vi "Autonomous Independent.vi"() -> ()   [LabVIEW 2014]
doc: "This VI is called when autonomous begins, and will automatically be terminated when autonomous ends. You can carry out timed or sensor driven robot movement independently without needing to return to the caller."
uses:
  <vilib>/Rock Robotics/WPI/Joystick/WPI_JoystickGetSetRefNum.vi
  <vilib>/Rock Robotics/WPI/RobotDrive/WPI_RobotDriveGetSetRefNum.vi
  <vilib>/Rock Robotics/WPI/RobotDrive/WPI_RobotDriveMecanumDrive_Cartesian.vi
  <vilib>/Rock Robotics/WPI/RobotDrive/WPI_RobotDriveArcadeDrive_Standard(NoSaturation).vi
panel:
  out "?":string
  out "Current Movement, for debugging 2":T1 {"Y Joystick Value" scale=1.0..-1.0; "X Joystick Value" scale=-1.0..1.0}
  in  "Array of robot movements 2":T2(array[cluster]) {"Y Joystick Value" scale=1.0..-1.0; "X Joystick Value" scale=-1.0..1.0}
  out "?":string
  out "Current Movement, for debugging":T1 {"Y Joystick Value" scale=1.0..-1.0; "X Joystick Value" scale=-1.0..1.0}
  in  "Array of robot movements":T2(array[cluster]) {"Y Joystick Value" scale=1.0..-1.0; "X Joystick Value" scale=-1.0..1.0}
  # "Be sure to right-click and choose Data Operations>>Make Current Value default if you want to save the array values with the VI"
  # "Be sure to right-click and choose Data Operations>>Make Current Value default if you want to save the array values with the VI"
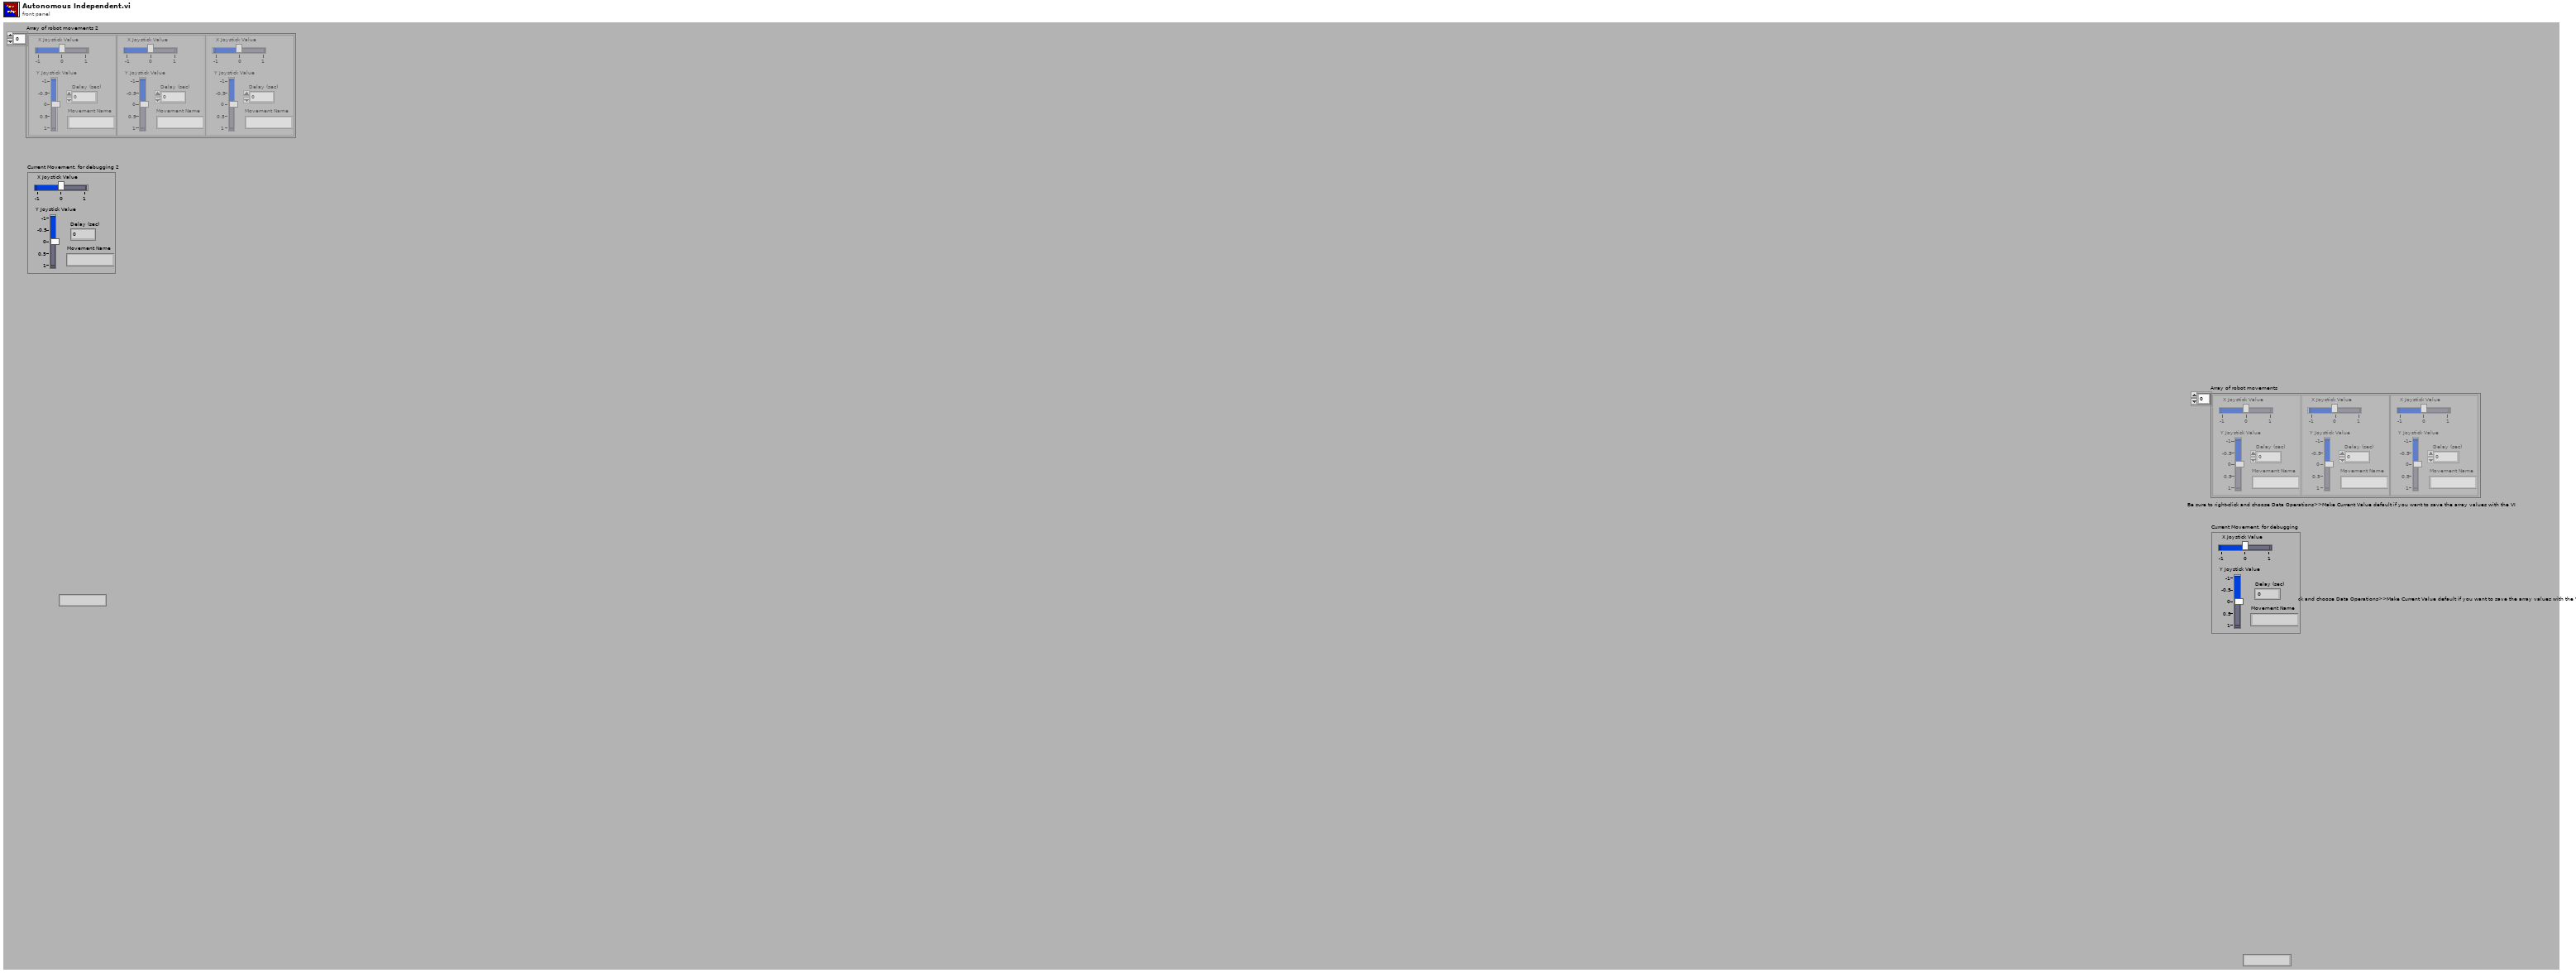
[diagram p1: front panel]
types:
  T1 = cluster{"X Joystick Value":dbl, "Y Joystick Value":dbl, "Delay (sec)":dbl, "Movement Name":string}
  T2 = cluster{"X Joystick Value":dbl, "Y Joystick Value":dbl, "Delay (sec)":dbl, "Movement Name":string}[]
  T3 = typedef "WPI_RobotDriveDevRef.ctl" = cluster{"DevStatus":errorcluster, "Motors[]":T4[], "Square Inputs":bool, "Max Output":dbl}
  T4 = typedef "WPI_MotorControlDeviceRef.ctl" = cluster{"DeviceStatus":errorcluster, "Type":T5, "PWM":cluster{"Controller":T6, "PWM Channel":T7, "DeadBand":T8}, "CAN":cluster{"Device Number":u8, "Control Mode":T9, "Semaphore":T10, "Max Vout":dbl, "TalonSRX Control Mode":T11}, "Invert":bool, "TransformRef":T12, "InvTransformRef":T12}
  T5 = typedef "WPI_MotorControlType.ctl" = enum16{"PWM", "CAN", "CANTalonSRX"}
  T6 = typedef "FPGA_TypedefDigitalModule.ctl" = enum16{"Controller 1"}
  T7 = typedef "FPGA_DIOPWMChannel.ctl" = enum8{"PWM 0", "PWM 1", "PWM 2", "PWM 3", "PWM 4", "PWM 5", "PWM 6", "PWM 7", "PWM 8", "PWM 9", "PWM MXP 0", "PWM MXP 1", "PWM MXP 2", "PWM MXP 3", "PWM MXP 4", "PWM MXP 5", "PWM MXP 6", "PWM MXP 7", "PWM MXP 8", "PWM MXP 9", "Invalid"}
  T8 = typedef "WPI_PWMDeadband.ctl" = cluster{"Name":string, "maxPositivePwm":i32, "minPositivePwm":i32, "centerPwm":i32, "maxNegativePwm":i32, "minNegativePwm":i32, "angularRange":u16}
  T9 = typedef "WPI_CANJaguar_ControlMode.ctl" = enum8{"Percent VBus", "Current", "Speed", "Position", "Voltage"}
  T10 = typedef "Semaphore RefNum" = refnum<k1>
  T11 = typedef "WPI_CANTalonSRX_APIControlMode.ctl" = enum8{"Percent VBus", "Speed", "Position", "Slave", "Unchanged / Invalid"}
  T12 = typedef "WPI_PWMTransform_ConPane.ctl" = refnum<vi>
  T13 = typedef "WPI_JoystickDevRef.ctl" = cluster{"Device":T14}
  T14 = typedef "WPI_JoystickDeviceEnum.ctl" = enum16{"USB 0", "USB 1", "USB 2", "USB 3", "USB 4", "USB 5"}
  T15 = cluster{"Rectangle":cluster{"Numeric":dbl, "Numeric 2":dbl, "Numeric 3":dbl, "Numeric 5":dbl}, "Scale %":dbl, "Score":dbl, "Correlation":dbl}[]
  T16 = cluster{"Distance (ft)":dbl, "Center":cluster{dbl, dbl}, "Normalized Rect":cluster{"Numeric":dbl, "Numeric 2":dbl, "Numeric 3":dbl, "Numeric 5":dbl}}[]
  T17 = cluster{"Rectangle":cluster{"Numeric":dbl, "Numeric 2":dbl, "Numeric 3":dbl, "Numeric 5":dbl}, "Scale %":dbl, "Score":dbl, "Correlation":dbl}
  T18 = cluster{"Distance (ft)":dbl, "Center":cluster{dbl, dbl}, "Normalized Rect":cluster{"Numeric":dbl, "Numeric 2":dbl, "Numeric 3":dbl, "Numeric 5":dbl}}
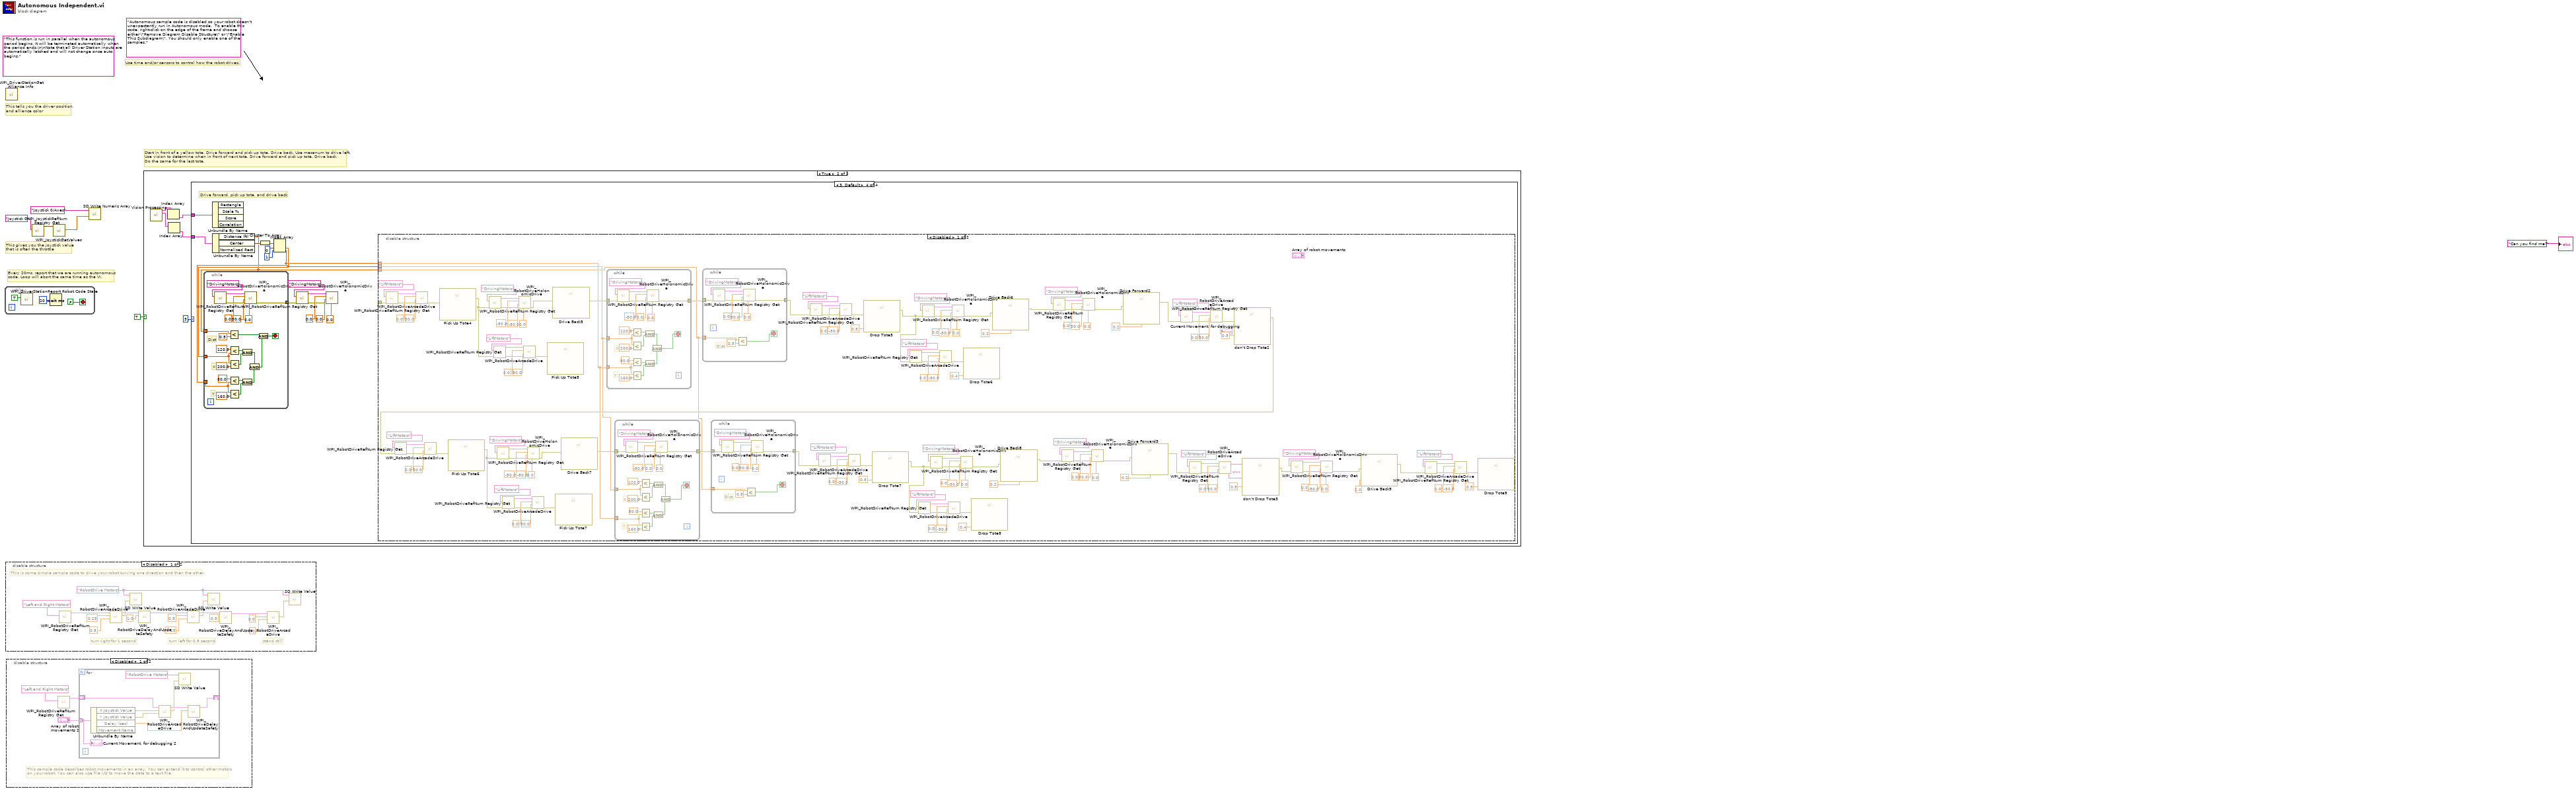
[diagram p0: block diagram]
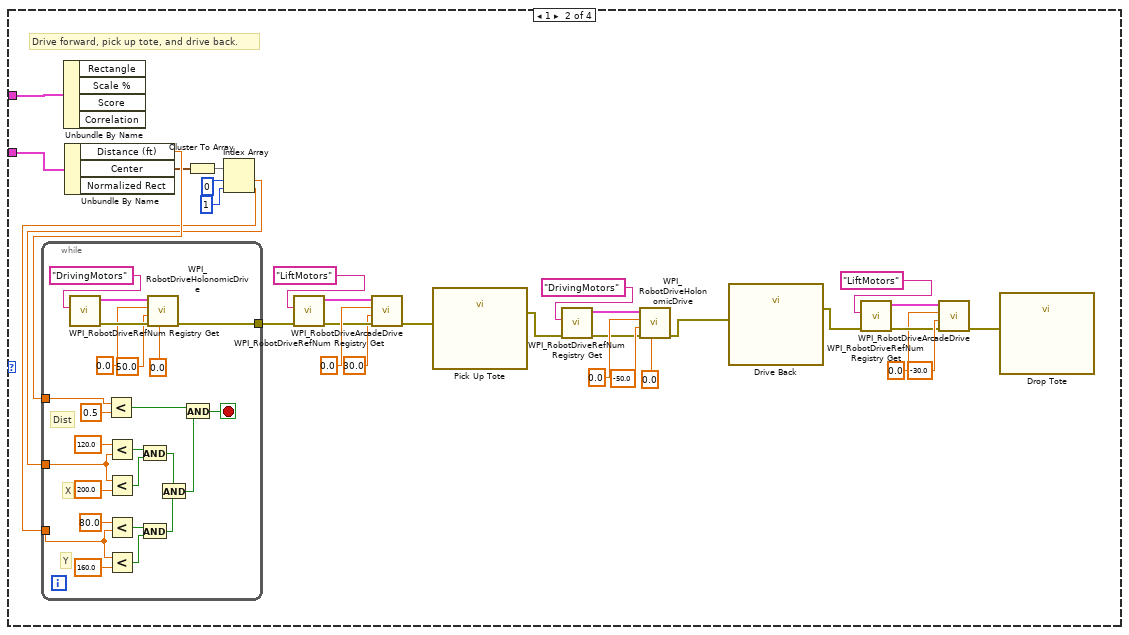
[diagram p4: hidden frame]
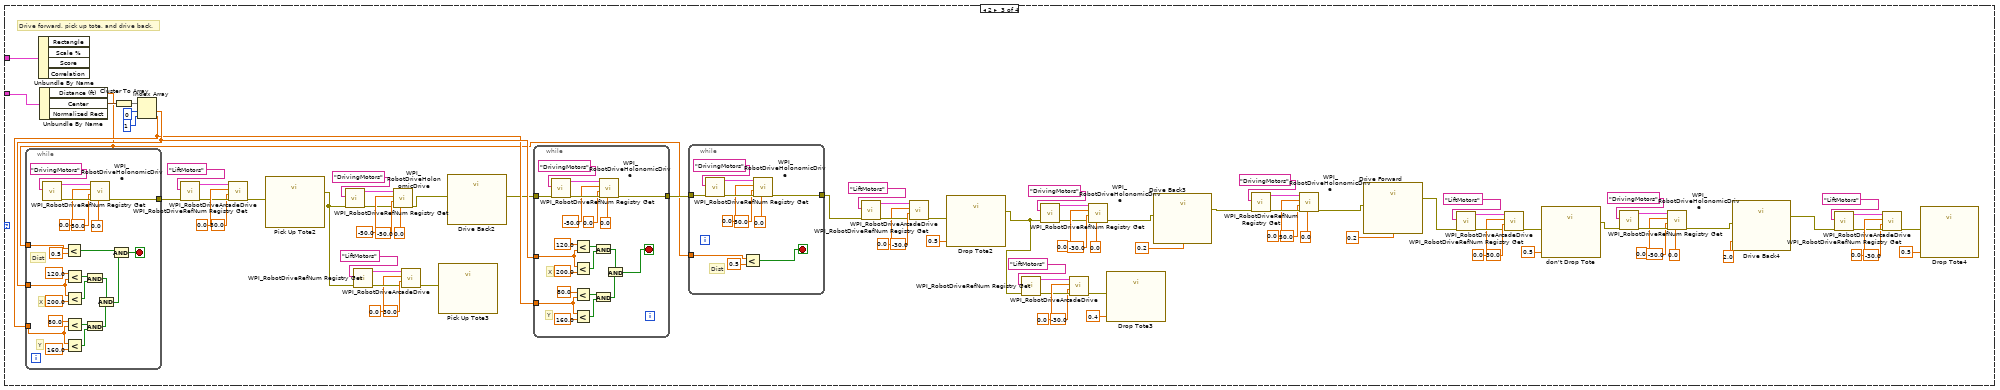
[diagram p5: hidden frame]
diagram:
  (unwired) "Autonomous sample code is disabled so your robot doesn't unexpectantly run in Autonomous mode.  To enable this code, right-click on the edge of the frame and choose either \"Remove Diagram Disable Structure\" or \"Enable This Subdiagram\". You should only enable one of the samples."
  (unwired) "This function is run in parallel when the autonomous period begins. It will be terminated automatically when the period ends.\n\nNote that all Driver Station inputs are automatically latched and will not change once auto begins."
  # "Start in front of a yellow tote. Drive forward and pick up tote. Drive back. Use mecanum to drive left.\nUse vision to determine when in front of next tote. Drive forward and pick up tote. Drive back.\nDo the same for the last tote."
  # "Every 20ms, report that we are running autonomous\ncode. Loop will abort the same time as the VI."
  # "This gives you the joystick value\nthat is often the throttle"
  # "Use time and/or sensors to control how the robot drives."
  # "This tells you the driver position\nand alliance color"
  n1 = while {
    stop <- FALSE stop-if-true
    n2 = call <vilib>:"WPI_DriverStationReport Robot Code State.vi"("Autonomous"=TRUE) -> ()  [unwired: 10 in, 1 out]
    n3 = Wait (ms)(milliseconds to wait=u32 20) -> ()  [unwired: 1 out]
  }
  n4 = call <vilib>:"WPI_DriverStationGet Alliance Info.vi"() -> ()  [unwired: 12 out]
  n5 = disable-structure shown="Disabled" {
    frame Disabled {
      w13 = "RobotDrive Motors" ("Name")
      # "This is some simple sample code to drive your robot curving one direction and then the other."
      # "stand still"
      # "turn left for 0.5 second"
      # "turn right for 1 second"
      n6 = call <vilib>:"WPI_RobotDriveRefNum Registry Get.vi"("refnum name"="Left and Right Motors") -> ("RobotDriveDevRef"=w14:T3)  [unwired: 1 in, 9 out]
      n7 = call-poly <vilib>:"WPI_RobotDriveArcadeDrive.vi"("Y axis value"=0.5 ("X axis value"), "X axis value"=0.25, "RobotDriveDevRef"=w14) -> ("Motor Values"=w12:dbl[], "RobotDriveDevRef"=w21:T3)  [unwired: 1 in, 6 out]
      n8 = call-poly <vilib>:"SD Write Value.vi"("Numeric Array"=w12, "Name"=w13) -> ()  [unwired: 8 in, 2 out]
      n9 = call <vilib>:"WPI_RobotDriveDelayAndUpdateSafety.vi"("Delay (s)"=1.0, "RobotDriveDevRef"=w21) -> ("RobotDriveDevRef 2"=w20:T3)  [unwired: 8 in, 1 out]
      n10 = call-poly <vilib>:"WPI_RobotDriveArcadeDrive.vi"("Y axis value"=0.25 ("X axis value"), "X axis value"=0.5, "RobotDriveDevRef"=w20) -> ("Motor Values"=w11:dbl[], "RobotDriveDevRef"=w19:T3)  [unwired: 1 in, 6 out]
      n11 = call-poly <vilib>:"SD Write Value.vi"("Numeric Array"=w11, "Name"=w13) -> ()  [unwired: 8 in, 2 out]
      n12 = call <vilib>:"WPI_RobotDriveDelayAndUpdateSafety.vi"("Delay (s)"=0.5, "RobotDriveDevRef"=w19) -> ("RobotDriveDevRef 2"=w18:T3)  [unwired: 8 in, 1 out]
      n13 = call-poly <vilib>:"WPI_RobotDriveArcadeDrive.vi"("Y axis value"=0.0 ("X axis value"), "X axis value"=0.0, "RobotDriveDevRef"=w18) -> ("Motor Values"=w10:dbl[])  [unwired: 1 in, 7 out]
      n14 = call-poly <vilib>:"SD Write Value.vi"("Numeric Array"=w10, "Name"=w13) -> ()  [unwired: 8 in, 2 out]
    }
    frame Enabled {
    }
  }
  n15 = disable-structure shown="Disabled" {
    frame Disabled {
      # "This sample code describes robot movements in an array. You can extend it to control other motors\non your robot. You can also use file I/O to move the data to a text file."
      n16 = call <vilib>:"WPI_RobotDriveRefNum Registry Get.vi"("refnum name"="Left and Right Motors") -> ("RobotDriveDevRef"=w29:T3)  [unwired: 1 in, 9 out]
      n17 = for {
        shift-right: [w36] -> _
        shift-left: w29 -> [w37]
        tunnel: "Array of robot movements 2" -> [w32] mode=indexing
        n18 = Unbundle By Name(w32) -> ("X Joystick Value"=w35:dbl, "Y Joystick Value"=w34:dbl, "Delay (sec)"=w33:dbl)  [unwired: 1 out]
        n19 = call-poly <vilib>:"WPI_RobotDriveArcadeDrive.vi"("Y axis value"=w34, "X axis value"=w35, "RobotDriveDevRef"=w37) -> ("Motor Values"=w31:dbl[], "RobotDriveDevRef"=w38:T3)  [unwired: 1 in, 6 out]
        n20 = call-poly <vilib>:"SD Write Value.vi"("Numeric Array"=w31, "Name"="RobotDrive Motors") -> ()  [unwired: 8 in, 2 out]
        n21 = call <vilib>:"WPI_RobotDriveDelayAndUpdateSafety.vi"("Delay (s)"=w33, "RobotDriveDevRef"=w38) -> ("RobotDriveDevRef 2"=w36:T3)  [unwired: 8 in, 1 out]
        "Current Movement, for debugging 2" <- w32
      }
    }
    frame Enabled {
    }
  }
  n22 = call <vilib>:"WPI_JoystickRefNum Registry Get.vi"("refnum name"="Joystick 0") -> ("JoystickDevRef"=w5:T13)  [unwired: 1 in, 9 out]
  n23 = call <vilib>:"WPI_JoystickGetValues.vi"("JoystickDevRef"=w5) -> ("Axes"=w3:dbl[])  [unwired: 6 in, 4 out]
  n24 = call <vilib>:"SD Write Numeric Array.vi"("Numeric Array"=w3, "Name"="Joystick 0/Axes") -> ()  [unwired: 8 in, 2 out]
  n25 = case shown="True" TRUE {
    frame False {
    }
    frame True {
      n26 = call "Vision Processing.vi"() -> ("Sorted Scores"=w41:T15, "Detected Totes"=w40:T16)  [unwired: 11 in, 3 out]
      n27 = Index Array(array=w41) -> (element=w43:T17)  [unwired: 1 in]
      n28 = Index Array(array=w40) -> (element=w42:T18)  [unwired: 1 in]
      n29 = case shown="3, Default" 3 {
        tunnel: w43 -> [_ w75 w189 w261]
        tunnel: w42 -> [_ w74 w188 w260]
        frame 0 {
        }
        frame 1 {
          # "Drive forward, pick up tote, and drive back."
          n30 = Unbundle By Name(w75) -> ()  [unwired: 4 out]
          n31 = Unbundle By Name(w74) -> ("Distance (ft)"=w73:dbl, "Center"=w71:cluster{dbl, dbl})  [unwired: 1 out]
          n32 = Cluster To Array(cluster=w71) -> (array=w72:dbl[])
          n33 = Index Array(array=w72, index #1=0 ("index"), index #2=1 ("index")) -> (element #1=w68:dbl, element #2=w67:dbl)
          n34 = while {
            tunnel: w73 -> [w92]
            tunnel: w68 -> [w91]
            tunnel: w67 -> [w82]
            tunnel: [w76] -> w62
            stop <- w77 stop-if-true
            # "Y"
            # "X"
            # "Dist"
            n35 = call <vilib>:"WPI_RobotDriveRefNum Registry Get.vi"("refnum name"="DrivingMotors") -> ("error out"=w97:errorcluster, "RobotDriveDevRef"=w99:T3)  [unwired: 9 in]
            n36 = Less?(x=w92, y=0.5) -> (x < y?=w79:bool)
            n37 = Less?(x=120.0, y=w91) -> (x < y?=w87:bool)
            n38 = Less?(x=w91, y=200.0) -> (x < y?=w88:bool)
            n39 = Less?(x=80.0, y=w82) -> (x < y?=w86:bool)
            n40 = Less?(x=w82, y=160.0) -> (x < y?=w85:bool)
            n41 = And(x=w87, y=w88) -> (x .and. y?=w80:bool)
            n42 = And(x=w86, y=w85) -> (x .and. y?=w81:bool)
            n43 = call-poly <vilib>:"WPI_RobotDriveHolonomicDrive.vi"("Rotation"=0.0, "error in (no error)"=w97, "Y"=50.0, "X"=0.0, "RobotDriveDevRef"=w99) -> ("error out"=w76:errorcluster)  [unwired: 4 in, 2 out]
            n44 = And(x=w80, y=w81) -> (x .and. y?=w78:bool)
            n45 = And(x=w79, y=w78) -> (x .and. y?=w77:bool)
          }
          n46 = call <vilib>:"WPI_RobotDriveRefNum Registry Get.vi"("error in (no error)"=w62, "refnum name"="LiftMotors") -> ("error out"=w65:errorcluster, "RobotDriveDevRef"=w63:T3)  [unwired: 8 in]
          n47 = call-poly <vilib>:"WPI_RobotDriveArcadeDrive.vi"("error in (no error)"=w65, "Y axis value"=30.0, "X axis value"=0.0 ("X"), "RobotDriveDevRef"=w63) -> ("error out"=w61:errorcluster)  [unwired: 5 in, 2 out]
          n48 = call "Pick Up Tote"("error in (no error)"=w61) -> ("error out"=w53:errorcluster)  [unwired: 10 in]
          n49 = call <vilib>:"WPI_RobotDriveRefNum Registry Get.vi"("error in (no error)"=w53, "refnum name"="DrivingMotors") -> ("error out"=w56:errorcluster, "RobotDriveDevRef"=w54:T3)  [unwired: 8 in]
          n50 = call-poly <vilib>:"WPI_RobotDriveHolonomicDrive.vi"("Rotation"=0.0, "error in (no error)"=w56, "Y"=-50.0, "X"=0.0, "RobotDriveDevRef"=w54) -> ("error out"=w52:errorcluster)  [unwired: 4 in, 2 out]
          n51 = call "Drive Back"("error in (no error)"=w52) -> ("error out"=w45:errorcluster)  [unwired: 10 in]
          n52 = call <vilib>:"WPI_RobotDriveRefNum Registry Get.vi"("error in (no error)"=w45, "refnum name"="LiftMotors") -> ("error out"=w47:errorcluster, "RobotDriveDevRef"=w49:T3)  [unwired: 8 in]
          n53 = call-poly <vilib>:"WPI_RobotDriveArcadeDrive.vi"("error in (no error)"=w47, "Y axis value"=-30.0, "X axis value"=0.0 ("X"), "RobotDriveDevRef"=w49) -> ("error out"=w50:errorcluster)  [unwired: 5 in, 2 out]
          n54 = call "Drop Tote"("error in (no error)"=w50) -> ()  [unwired: 10 in, 1 out]
        }
        frame 2 {
          # "Drive forward, pick up tote, and drive back."
          n55 = Unbundle By Name(w189) -> ()  [unwired: 4 out]
          n56 = Unbundle By Name(w188) -> ("Distance (ft)"=w159:dbl, "Center"=w186:cluster{dbl, dbl})  [unwired: 1 out]
          n57 = Cluster To Array(cluster=w186) -> (array=w187:dbl[])
          n58 = Index Array(array=w187, index #1=0 ("index"), index #2=1 ("index")) -> (element #1=w163:dbl, element #2=w162:dbl)
          n59 = while {
            tunnel: w159 -> [w238]
            tunnel: w163 -> [w237]
            tunnel: w162 -> [w228]
            tunnel: [w222] -> w179
            stop <- w223 stop-if-true
            # "Y"
            # "X"
            # "Dist"
            n60 = call <vilib>:"WPI_RobotDriveRefNum Registry Get.vi"("refnum name"="DrivingMotors") -> ("error out"=w243:errorcluster, "RobotDriveDevRef"=w245:T3)  [unwired: 9 in]
            n61 = Less?(x=w238, y=0.5) -> (x < y?=w225:bool)
            n62 = Less?(x=120.0, y=w237) -> (x < y?=w233:bool)
            n63 = Less?(x=w237, y=200.0) -> (x < y?=w234:bool)
            n64 = Less?(x=80.0, y=w228) -> (x < y?=w232:bool)
            n65 = Less?(x=w228, y=160.0) -> (x < y?=w231:bool)
            n66 = And(x=w233, y=w234) -> (x .and. y?=w226:bool)
            n67 = And(x=w232, y=w231) -> (x .and. y?=w227:bool)
            n68 = call-poly <vilib>:"WPI_RobotDriveHolonomicDrive.vi"("Rotation"=0.0, "error in (no error)"=w243, "Y"=50.0, "X"=0.0, "RobotDriveDevRef"=w245) -> ("error out"=w222:errorcluster)  [unwired: 4 in, 2 out]
            n69 = And(x=w226, y=w227) -> (x .and. y?=w224:bool)
            n70 = And(x=w225, y=w224) -> (x .and. y?=w223:bool)
          }
          n71 = call <vilib>:"WPI_RobotDriveRefNum Registry Get.vi"("error in (no error)"=w179, "refnum name"="LiftMotors") -> ("error out"=w182:errorcluster, "RobotDriveDevRef"=w180:T3)  [unwired: 8 in]
          n72 = call-poly <vilib>:"WPI_RobotDriveArcadeDrive.vi"("error in (no error)"=w182, "Y axis value"=30.0, "X axis value"=0.0 ("X"), "RobotDriveDevRef"=w180) -> ("error out"=w178:errorcluster)  [unwired: 5 in, 2 out]
          n73 = call "Pick Up Tote2"("error in (no error)"=w178) -> ("error out"=w152:errorcluster)  [unwired: 10 in]
          n74 = call <vilib>:"WPI_RobotDriveRefNum Registry Get.vi"("error in (no error)"=w152, "refnum name"="DrivingMotors") -> ("error out"=w173:errorcluster, "RobotDriveDevRef"=w171:T3)  [unwired: 8 in]
          n75 = call <vilib>:"WPI_RobotDriveRefNum Registry Get.vi"("error in (no error)"=w152, "refnum name"="LiftMotors") -> ("error out"=w154:errorcluster, "RobotDriveDevRef"=w156:T3)  [unwired: 8 in]
          n76 = call-poly <vilib>:"WPI_RobotDriveHolonomicDrive.vi"("Rotation"=0.0, "error in (no error)"=w173, "Y"=-50.0, "X"=-50.0, "RobotDriveDevRef"=w171) -> ("error out"=w170:errorcluster)  [unwired: 4 in, 2 out]
          n77 = call-poly <vilib>:"WPI_RobotDriveArcadeDrive.vi"("error in (no error)"=w154, "Y axis value"=30.0, "X axis value"=0.0 ("X"), "RobotDriveDevRef"=w156) -> ("error out"=w157:errorcluster)  [unwired: 5 in, 2 out]
          n78 = call "Pick Up Tote3"("error in (no error)"=w157) -> ()  [unwired: 10 in, 1 out]
          n79 = call "Drive Back2"("error in (no error)"=w170) -> ("error out"=w161:errorcluster)  [unwired: 10 in]
          n80 = while {
            tunnel: w163 -> [w215]
            tunnel: w162 -> [w206]
            tunnel: [w203] -> w160
            tunnel: w161 -> [w202]
            stop <- w201 stop-if-true
            # "Y"
            # "X"
            n81 = call <vilib>:"WPI_RobotDriveRefNum Registry Get.vi"("error in (no error)"=w202, "refnum name"="DrivingMotors") -> ("error out"=w219:errorcluster, "RobotDriveDevRef"=w221:T3)  [unwired: 8 in]
            n82 = Less?(x=120.0, y=w215) -> (x < y?=w211:bool)
            n83 = Less?(x=w215, y=200.0) -> (x < y?=w212:bool)
            n84 = Less?(x=80.0, y=w206) -> (x < y?=w210:bool)
            n85 = Less?(x=w206, y=160.0) -> (x < y?=w209:bool)
            n86 = And(x=w211, y=w212) -> (x .and. y?=w204:bool)
            n87 = And(x=w210, y=w209) -> (x .and. y?=w205:bool)
            n88 = call-poly <vilib>:"WPI_RobotDriveHolonomicDrive.vi"("Rotation"=0.0, "error in (no error)"=w219, "Y"=0.0, "X"=-50.0, "RobotDriveDevRef"=w221) -> ("error out"=w203:errorcluster)  [unwired: 4 in, 2 out]
            n89 = And(x=w204, y=w205) -> (x .and. y?=w201:bool)
          }
          n90 = while {
            tunnel: [w194] -> w151
            tunnel: w160 -> [w193]
            tunnel: w159 -> [w191]
            stop <- w190 stop-if-true
            # "Dist"
            n91 = call <vilib>:"WPI_RobotDriveRefNum Registry Get.vi"("error in (no error)"=w193, "refnum name"="DrivingMotors") -> ("error out"=w198:errorcluster, "RobotDriveDevRef"=w200:T3)  [unwired: 8 in]
            n92 = Less?(x=w191, y=0.5) -> (x < y?=w190:bool)
            n93 = call-poly <vilib>:"WPI_RobotDriveHolonomicDrive.vi"("Rotation"=0.0, "error in (no error)"=w198, "Y"=50.0, "X"=0.0, "RobotDriveDevRef"=w200) -> ("error out"=w194:errorcluster)  [unwired: 4 in, 2 out]
          }
          n94 = call <vilib>:"WPI_RobotDriveRefNum Registry Get.vi"("error in (no error)"=w151, "refnum name"="LiftMotors") -> ("error out"=w165:errorcluster, "RobotDriveDevRef"=w167:T3)  [unwired: 8 in]
          n95 = call-poly <vilib>:"WPI_RobotDriveArcadeDrive.vi"("error in (no error)"=w165, "Y axis value"=-30.0, "X axis value"=0.0 ("X"), "RobotDriveDevRef"=w167) -> ("error out"=w168:errorcluster)  [unwired: 5 in, 2 out]
          n96 = call "Drop Tote2"("error in (no error)"=w168, "Delay Time (s)"=0.5) -> ("error out"=w134:errorcluster)  [unwired: 9 in]
          n97 = call <vilib>:"WPI_RobotDriveRefNum Registry Get.vi"("error in (no error)"=w134, "refnum name"="LiftMotors") -> ("error out"=w139:errorcluster, "RobotDriveDevRef"=w137:T3)  [unwired: 8 in]
          n98 = call <vilib>:"WPI_RobotDriveRefNum Registry Get.vi"("error in (no error)"=w134, "refnum name"="DrivingMotors") -> ("error out"=w146:errorcluster, "RobotDriveDevRef"=w144:T3)  [unwired: 8 in]
          n99 = call-poly <vilib>:"WPI_RobotDriveArcadeDrive.vi"("error in (no error)"=w139, "Y axis value"=-30.0, "X axis value"=0.0 ("X"), "RobotDriveDevRef"=w137) -> ("error out"=w136:errorcluster)  [unwired: 5 in, 2 out]
          n100 = call-poly <vilib>:"WPI_RobotDriveHolonomicDrive.vi"("Rotation"=0.0, "error in (no error)"=w146, "Y"=-30.0, "X"=0.0, "RobotDriveDevRef"=w144) -> ("error out"=w143:errorcluster)  [unwired: 4 in, 2 out]
          n101 = call "Drop Tote3"("error in (no error)"=w136, "Delay Time (s)"=0.4) -> ()  [unwired: 9 in, 1 out]
          n102 = call "Drive Back3"("error in (no error)"=w143, "Delay Time (s)"=0.2) -> ("error out"=w125:errorcluster)  [unwired: 9 in]
          n103 = call <vilib>:"WPI_RobotDriveRefNum Registry Get.vi"("error in (no error)"=w125, "refnum name"="DrivingMotors") -> ("error out"=w129:errorcluster, "RobotDriveDevRef"=w131:T3)  [unwired: 8 in]
          n104 = call-poly <vilib>:"WPI_RobotDriveHolonomicDrive.vi"("Rotation"=0.0, "error in (no error)"=w129, "Y"=30.0, "X"=0.0, "RobotDriveDevRef"=w131) -> ("error out"=w132:errorcluster)  [unwired: 4 in, 2 out]
          n105 = call "Drive Forward"("error in (no error)"=w132, "Delay Time (s)"=0.2) -> ("error out"=w117:errorcluster)  [unwired: 9 in]
          n106 = call <vilib>:"WPI_RobotDriveRefNum Registry Get.vi"("error in (no error)"=w117, "refnum name"="LiftMotors") -> ("error out"=w120:errorcluster, "RobotDriveDevRef"=w122:T3)  [unwired: 8 in]
          n107 = call-poly <vilib>:"WPI_RobotDriveArcadeDrive.vi"("error in (no error)"=w120, "Y axis value"=30.0, "X axis value"=0.0 ("X"), "RobotDriveDevRef"=w122) -> ("error out"=w123:errorcluster)  [unwired: 5 in, 2 out]
          n108 = call "don't Drop Tote"("error in (no error)"=w123, "Delay Time (s)"=0.5) -> ("error out"=w109:errorcluster)  [unwired: 9 in]
          n109 = call <vilib>:"WPI_RobotDriveRefNum Registry Get.vi"("error in (no error)"=w109, "refnum name"="DrivingMotors") -> ("error out"=w113:errorcluster, "RobotDriveDevRef"=w115:T3)  [unwired: 8 in]
          n110 = call-poly <vilib>:"WPI_RobotDriveHolonomicDrive.vi"("Rotation"=0.0, "error in (no error)"=w113, "Y"=-50.0, "X"=0.0, "RobotDriveDevRef"=w115) -> ("error out"=w116:errorcluster)  [unwired: 4 in, 2 out]
          n111 = call "Drive Back4"("error in (no error)"=w116, "Delay Time (s)"=2.0) -> ("error out"=w100:errorcluster)  [unwired: 9 in]
          n112 = call <vilib>:"WPI_RobotDriveRefNum Registry Get.vi"("error in (no error)"=w100, "refnum name"="LiftMotors") -> ("error out"=w105:errorcluster, "RobotDriveDevRef"=w103:T3)  [unwired: 8 in]
          n113 = call-poly <vilib>:"WPI_RobotDriveArcadeDrive.vi"("error in (no error)"=w105, "Y axis value"=-30.0, "X axis value"=0.0 ("X"), "RobotDriveDevRef"=w103) -> ("error out"=w102:errorcluster)  [unwired: 5 in, 2 out]
          n114 = call "Drop Tote4"("error in (no error)"=w102, "Delay Time (s)"=0.5) -> ()  [unwired: 9 in, 1 out]
        }
        frame 3, Default {
          # "Drive forward, pick up tote, and drive back."
          n115 = Unbundle By Name(w261) -> ()  [unwired: 4 out]
          n116 = Unbundle By Name(w260) -> ("Distance (ft)"=w253:dbl, "Center"=w258:cluster{dbl, dbl})  [unwired: 1 out]
          n117 = Cluster To Array(cluster=w258) -> (array=w259:dbl[])
          n118 = Index Array(array=w259, index #1=0 ("index"), index #2=1 ("index")) -> (element #1=w255:dbl, element #2=w254:dbl)
          n119 = while {
            tunnel: w253 -> [w490]
            tunnel: w255 -> [w489]
            tunnel: w254 -> [w480]
            tunnel: [w474] -> w246
            stop <- w475 stop-if-true
            # "Y"
            # "X"
            # "Dist"
            n120 = call <vilib>:"WPI_RobotDriveRefNum Registry Get.vi"("refnum name"="DrivingMotors") -> ("error out"=w495:errorcluster, "RobotDriveDevRef"=w497:T3)  [unwired: 9 in]
            n121 = Less?(x=w490, y=0.5) -> (x < y?=w477:bool)
            n122 = Less?(x=120.0, y=w489) -> (x < y?=w485:bool)
            n123 = Less?(x=w489, y=200.0) -> (x < y?=w486:bool)
            n124 = Less?(x=80.0, y=w480) -> (x < y?=w484:bool)
            n125 = Less?(x=w480, y=160.0) -> (x < y?=w483:bool)
            n126 = And(x=w485, y=w486) -> (x .and. y?=w478:bool)
            n127 = And(x=w484, y=w483) -> (x .and. y?=w479:bool)
            n128 = call-poly <vilib>:"WPI_RobotDriveHolonomicDrive.vi"("Rotation"=0.0, "error in (no error)"=w495, "Y"=50.0, "X"=0.0, "RobotDriveDevRef"=w497) -> ("error out"=w474:errorcluster)  [unwired: 4 in, 2 out]
            n129 = And(x=w478, y=w479) -> (x .and. y?=w476:bool)
            n130 = And(x=w477, y=w476) -> (x .and. y?=w475:bool)
          }
          n131 = call <vilib>:"WPI_RobotDriveRefNum Registry Get.vi"("error in (no error)"=w246, "refnum name"="DrivingMotors") -> ("error out"=w249:errorcluster, "RobotDriveDevRef"=w247:T3)  [unwired: 8 in]
          n132 = call-poly <vilib>:"WPI_RobotDriveHolonomicDrive.vi"("Rotation"=0.0, "error in (no error)"=w249, "Y"=0.0, "X"=0.0, "RobotDriveDevRef"=w247) -> ()  [unwired: 4 in, 3 out]
          n133 = disable-structure shown="Disabled" {
            disable-tunnel: _ -> [w405 _]
            disable-tunnel: w255 -> [w264 _]
            disable-tunnel: w254 -> [w263 _]
            disable-tunnel: w253 -> [w262 _]
            frame Disabled {
              n134 = call <vilib>:"WPI_RobotDriveRefNum Registry Get.vi"("error in (no error)"=w405, "refnum name"="LiftMotors") -> ("error out"=w408:errorcluster, "RobotDriveDevRef"=w406:T3)  [unwired: 8 in]
              n135 = call-poly <vilib>:"WPI_RobotDriveArcadeDrive.vi"("error in (no error)"=w408, "Y axis value"=30.0, "X axis value"=0.0 ("X"), "RobotDriveDevRef"=w406) -> ("error out"=w404:errorcluster)  [unwired: 5 in, 2 out]
              n136 = call "Pick Up Tote4"("error in (no error)"=w404) -> ("error out"=w381:errorcluster)  [unwired: 10 in]
              n137 = call <vilib>:"WPI_RobotDriveRefNum Registry Get.vi"("error in (no error)"=w381, "refnum name"="DrivingMotors") -> ("error out"=w399:errorcluster, "RobotDriveDevRef"=w397:T3)  [unwired: 8 in]
              n138 = call <vilib>:"WPI_RobotDriveRefNum Registry Get.vi"("error in (no error)"=w381, "refnum name"="LiftMotors") -> ("error out"=w383:errorcluster, "RobotDriveDevRef"=w385:T3)  [unwired: 8 in]
              n139 = call-poly <vilib>:"WPI_RobotDriveHolonomicDrive.vi"("Rotation"=0.0, "error in (no error)"=w399, "Y"=-50.0, "X"=-50.0, "RobotDriveDevRef"=w397) -> ("error out"=w396:errorcluster)  [unwired: 4 in, 2 out]
              n140 = call-poly <vilib>:"WPI_RobotDriveArcadeDrive.vi"("error in (no error)"=w383, "Y axis value"=30.0, "X axis value"=0.0 ("X"), "RobotDriveDevRef"=w385) -> ("error out"=w386:errorcluster)  [unwired: 5 in, 2 out]
              n141 = call "Pick Up Tote5"("error in (no error)"=w386) -> ()  [unwired: 10 in, 1 out]
              n142 = call "Drive Back5"("error in (no error)"=w396) -> ("error out"=w389:errorcluster)  [unwired: 10 in]
              n143 = while {
                tunnel: w264 -> [w446]
                tunnel: w263 -> [w437]
                tunnel: [w434] -> w388
                tunnel: w389 -> [w433]
                stop <- w432 stop-if-true
                # "Y"
                # "X"
                n144 = call <vilib>:"WPI_RobotDriveRefNum Registry Get.vi"("error in (no error)"=w433, "refnum name"="DrivingMotors") -> ("error out"=w450:errorcluster, "RobotDriveDevRef"=w452:T3)  [unwired: 8 in]
                n145 = Less?(x=120.0, y=w446) -> (x < y?=w442:bool)
                n146 = Less?(x=w446, y=200.0) -> (x < y?=w443:bool)
                n147 = Less?(x=80.0, y=w437) -> (x < y?=w441:bool)
                n148 = Less?(x=w437, y=160.0) -> (x < y?=w440:bool)
                n149 = And(x=w442, y=w443) -> (x .and. y?=w435:bool)
                n150 = And(x=w441, y=w440) -> (x .and. y?=w436:bool)
                n151 = call-poly <vilib>:"WPI_RobotDriveHolonomicDrive.vi"("Rotation"=0.0, "error in (no error)"=w450, "Y"=0.0, "X"=-50.0, "RobotDriveDevRef"=w452) -> ("error out"=w434:errorcluster)  [unwired: 4 in, 2 out]
                n152 = And(x=w435, y=w436) -> (x .and. y?=w432:bool)
              }
              n153 = while {
                tunnel: [w425] -> w380
                tunnel: w388 -> [w424]
                tunnel: w262 -> [w422]
                stop <- w421 stop-if-true
                # "Dist"
                n154 = call <vilib>:"WPI_RobotDriveRefNum Registry Get.vi"("error in (no error)"=w424, "refnum name"="DrivingMotors") -> ("error out"=w429:errorcluster, "RobotDriveDevRef"=w431:T3)  [unwired: 8 in]
                n155 = Less?(x=w422, y=0.5) -> (x < y?=w421:bool)
                n156 = call-poly <vilib>:"WPI_RobotDriveHolonomicDrive.vi"("Rotation"=0.0, "error in (no error)"=w429, "Y"=50.0, "X"=0.0, "RobotDriveDevRef"=w431) -> ("error out"=w425:errorcluster)  [unwired: 4 in, 2 out]
              }
              n157 = call <vilib>:"WPI_RobotDriveRefNum Registry Get.vi"("error in (no error)"=w380, "refnum name"="LiftMotors") -> ("error out"=w391:errorcluster, "RobotDriveDevRef"=w393:T3)  [unwired: 8 in]
              n158 = call-poly <vilib>:"WPI_RobotDriveArcadeDrive.vi"("error in (no error)"=w391, "Y axis value"=-30.0, "X axis value"=0.0 ("X"), "RobotDriveDevRef"=w393) -> ("error out"=w394:errorcluster)  [unwired: 5 in, 2 out]
              n159 = call "Drop Tote5"("error in (no error)"=w394, "Delay Time (s)"=0.5) -> ("error out"=w363:errorcluster)  [unwired: 9 in]
              n160 = call <vilib>:"WPI_RobotDriveRefNum Registry Get.vi"("error in (no error)"=w363, "refnum name"="LiftMotors") -> ("error out"=w368:errorcluster, "RobotDriveDevRef"=w366:T3)  [unwired: 8 in]
              n161 = call <vilib>:"WPI_RobotDriveRefNum Registry Get.vi"("error in (no error)"=w363, "refnum name"="DrivingMotors") -> ("error out"=w375:errorcluster, "RobotDriveDevRef"=w373:T3)  [unwired: 8 in]
              n162 = call-poly <vilib>:"WPI_RobotDriveArcadeDrive.vi"("error in (no error)"=w368, "Y axis value"=-30.0, "X axis value"=0.0 ("X"), "RobotDriveDevRef"=w366) -> ("error out"=w365:errorcluster)  [unwired: 5 in, 2 out]
              n163 = call-poly <vilib>:"WPI_RobotDriveHolonomicDrive.vi"("Rotation"=0.0, "error in (no error)"=w375, "Y"=-30.0, "X"=0.0, "RobotDriveDevRef"=w373) -> ("error out"=w372:errorcluster)  [unwired: 4 in, 2 out]
              n164 = call "Drop Tote6"("error in (no error)"=w365, "Delay Time (s)"=0.4) -> ()  [unwired: 9 in, 1 out]
              n165 = call "Drive Back6"("error in (no error)"=w372, "Delay Time (s)"=0.2) -> ("error out"=w354:errorcluster)  [unwired: 9 in]
              n166 = call <vilib>:"WPI_RobotDriveRefNum Registry Get.vi"("error in (no error)"=w354, "refnum name"="DrivingMotors") -> ("error out"=w358:errorcluster, "RobotDriveDevRef"=w360:T3)  [unwired: 8 in]
              n167 = call-poly <vilib>:"WPI_RobotDriveHolonomicDrive.vi"("Rotation"=0.0, "error in (no error)"=w358, "Y"=30.0, "X"=0.0, "RobotDriveDevRef"=w360) -> ("error out"=w361:errorcluster)  [unwired: 4 in, 2 out]
              n168 = call "Drive Forward2"("error in (no error)"=w361, "Delay Time (s)"=0.2) -> ("error out"=w346:errorcluster)  [unwired: 9 in]
              n169 = call <vilib>:"WPI_RobotDriveRefNum Registry Get.vi"("error in (no error)"=w346, "refnum name"="LiftMotors") -> ("error out"=w349:errorcluster, "RobotDriveDevRef"=w351:T3)  [unwired: 8 in]
              n170 = call-poly <vilib>:"WPI_RobotDriveArcadeDrive.vi"("error in (no error)"=w349, "Y axis value"=30.0, "X axis value"=0.0 ("X"), "RobotDriveDevRef"=w351) -> ("error out"=w352:errorcluster)  [unwired: 5 in, 2 out]
              n171 = call "don't Drop Tote2"("error in (no error)"=w352, "Delay Time (s)"=0.5) -> ("error out"=w265:errorcluster)  [unwired: 9 in]
              n172 = call <vilib>:"WPI_RobotDriveRefNum Registry Get.vi"("error in (no error)"=w265, "refnum name"="LiftMotors") -> ("error out"=w268:errorcluster, "RobotDriveDevRef"=w270:T3)  [unwired: 8 in]
              n173 = call-poly <vilib>:"WPI_RobotDriveArcadeDrive.vi"("error in (no error)"=w268, "Y axis value"=30.0, "X axis value"=0.0 ("X"), "RobotDriveDevRef"=w270) -> ("error out"=w271:errorcluster)  [unwired: 5 in, 2 out]
              n174 = call "Pick Up Tote6"("error in (no error)"=w271) -> ("error out"=w294:errorcluster)  [unwired: 10 in]
              n175 = call <vilib>:"WPI_RobotDriveRefNum Registry Get.vi"("error in (no error)"=w294, "refnum name"="DrivingMotors") -> ("error out"=w276:errorcluster, "RobotDriveDevRef"=w278:T3)  [unwired: 8 in]
              n176 = call <vilib>:"WPI_RobotDriveRefNum Registry Get.vi"("error in (no error)"=w294, "refnum name"="LiftMotors") -> ("error out"=w292:errorcluster, "RobotDriveDevRef"=w290:T3)  [unwired: 8 in]
              n177 = call-poly <vilib>:"WPI_RobotDriveHolonomicDrive.vi"("Rotation"=0.0, "error in (no error)"=w276, "Y"=-50.0, "X"=-50.0, "RobotDriveDevRef"=w278) -> ("error out"=w279:errorcluster)  [unwired: 4 in, 2 out]
              n178 = call-poly <vilib>:"WPI_RobotDriveArcadeDrive.vi"("error in (no error)"=w292, "Y axis value"=30.0, "X axis value"=0.0 ("X"), "RobotDriveDevRef"=w290) -> ("error out"=w289:errorcluster)  [unwired: 5 in, 2 out]
              n179 = call "Pick Up Tote7"("error in (no error)"=w289) -> ()  [unwired: 10 in, 1 out]
              n180 = call "Drive Back7"("error in (no error)"=w279) -> ("error out"=w286:errorcluster)  [unwired: 10 in]
              n181 = while {
                tunnel: w264 -> [w467]
                tunnel: w263 -> [w458]
                tunnel: [w455] -> w287
                tunnel: w286 -> [w454]
                stop <- w453 stop-if-true
                # "Y"
                # "X"
                n182 = call <vilib>:"WPI_RobotDriveRefNum Registry Get.vi"("error in (no error)"=w454, "refnum name"="DrivingMotors") -> ("error out"=w471:errorcluster, "RobotDriveDevRef"=w473:T3)  [unwired: 8 in]
                n183 = Less?(x=120.0, y=w467) -> (x < y?=w463:bool)
                n184 = Less?(x=w467, y=200.0) -> (x < y?=w464:bool)
                n185 = Less?(x=80.0, y=w458) -> (x < y?=w462:bool)
                n186 = Less?(x=w458, y=160.0) -> (x < y?=w461:bool)
                n187 = And(x=w463, y=w464) -> (x .and. y?=w456:bool)
                n188 = And(x=w462, y=w461) -> (x .and. y?=w457:bool)
                n189 = call-poly <vilib>:"WPI_RobotDriveHolonomicDrive.vi"("Rotation"=0.0, "error in (no error)"=w471, "Y"=0.0, "X"=-50.0, "RobotDriveDevRef"=w473) -> ("error out"=w455:errorcluster)  [unwired: 4 in, 2 out]
                n190 = And(x=w456, y=w457) -> (x .and. y?=w453:bool)
              }
              n191 = while {
                tunnel: [w414] -> w295
                tunnel: w287 -> [w413]
                tunnel: w262 -> [w411]
                stop <- w410 stop-if-true
                # "Dist"
                n192 = call <vilib>:"WPI_RobotDriveRefNum Registry Get.vi"("error in (no error)"=w413, "refnum name"="DrivingMotors") -> ("error out"=w418:errorcluster, "RobotDriveDevRef"=w420:T3)  [unwired: 8 in]
                n193 = Less?(x=w411, y=0.5) -> (x < y?=w410:bool)
                n194 = call-poly <vilib>:"WPI_RobotDriveHolonomicDrive.vi"("Rotation"=0.0, "error in (no error)"=w418, "Y"=50.0, "X"=0.0, "RobotDriveDevRef"=w420) -> ("error out"=w414:errorcluster)  [unwired: 4 in, 2 out]
              }
              n195 = call <vilib>:"WPI_RobotDriveRefNum Registry Get.vi"("error in (no error)"=w295, "refnum name"="LiftMotors") -> ("error out"=w284:errorcluster, "RobotDriveDevRef"=w282:T3)  [unwired: 8 in]
              n196 = call-poly <vilib>:"WPI_RobotDriveArcadeDrive.vi"("error in (no error)"=w284, "Y axis value"=-30.0, "X axis value"=0.0 ("X"), "RobotDriveDevRef"=w282) -> ("error out"=w281:errorcluster)  [unwired: 5 in, 2 out]
              n197 = call "Drop Tote7"("error in (no error)"=w281, "Delay Time (s)"=0.5) -> ("error out"=w312:errorcluster)  [unwired: 9 in]
              n198 = call <vilib>:"WPI_RobotDriveRefNum Registry Get.vi"("error in (no error)"=w312, "refnum name"="LiftMotors") -> ("error out"=w307:errorcluster, "RobotDriveDevRef"=w309:T3)  [unwired: 8 in]
              n199 = call <vilib>:"WPI_RobotDriveRefNum Registry Get.vi"("error in (no error)"=w312, "refnum name"="DrivingMotors") -> ("error out"=w300:errorcluster, "RobotDriveDevRef"=w302:T3)  [unwired: 8 in]
              n200 = call-poly <vilib>:"WPI_RobotDriveArcadeDrive.vi"("error in (no error)"=w307, "Y axis value"=-30.0, "X axis value"=0.0 ("X"), "RobotDriveDevRef"=w309) -> ("error out"=w310:errorcluster)  [unwired: 5 in, 2 out]
              n201 = call-poly <vilib>:"WPI_RobotDriveHolonomicDrive.vi"("Rotation"=0.0, "error in (no error)"=w300, "Y"=-30.0, "X"=0.0, "RobotDriveDevRef"=w302) -> ("error out"=w303:errorcluster)  [unwired: 4 in, 2 out]
              n202 = call "Drop Tote8"("error in (no error)"=w310, "Delay Time (s)"=0.4) -> ()  [unwired: 9 in, 1 out]
              n203 = call "Drive Back8"("error in (no error)"=w303, "Delay Time (s)"=0.2) -> ("error out"=w321:errorcluster)  [unwired: 9 in]
              n204 = call <vilib>:"WPI_RobotDriveRefNum Registry Get.vi"("error in (no error)"=w321, "refnum name"="DrivingMotors") -> ("error out"=w317:errorcluster, "RobotDriveDevRef"=w315:T3)  [unwired: 8 in]
              n205 = call-poly <vilib>:"WPI_RobotDriveHolonomicDrive.vi"("Rotation"=0.0, "error in (no error)"=w317, "Y"=30.0, "X"=0.0, "RobotDriveDevRef"=w315) -> ("error out"=w314:errorcluster)  [unwired: 4 in, 2 out]
              n206 = call "Drive Forward3"("error in (no error)"=w314, "Delay Time (s)"=0.2) -> ("error out"=w329:errorcluster)  [unwired: 9 in]
              n207 = call <vilib>:"WPI_RobotDriveRefNum Registry Get.vi"("error in (no error)"=w329, "refnum name"="LiftMotors") -> ("error out"=w326:errorcluster, "RobotDriveDevRef"=w324:T3)  [unwired: 8 in]
              n208 = call-poly <vilib>:"WPI_RobotDriveArcadeDrive.vi"("error in (no error)"=w326, "Y axis value"=30.0, "X axis value"=0.0 ("X"), "RobotDriveDevRef"=w324) -> ("error out"=w323:errorcluster)  [unwired: 5 in, 2 out]
              n209 = call "don't Drop Tote3"("error in (no error)"=w323, "Delay Time (s)"=0.5) -> ("error out"=w337:errorcluster)  [unwired: 9 in]
              n210 = call <vilib>:"WPI_RobotDriveRefNum Registry Get.vi"("error in (no error)"=w337, "refnum name"="DrivingMotors") -> ("error out"=w333:errorcluster, "RobotDriveDevRef"=w331:T3)  [unwired: 8 in]
              n211 = call-poly <vilib>:"WPI_RobotDriveHolonomicDrive.vi"("Rotation"=0.0, "error in (no error)"=w333, "Y"=-50.0, "X"=0.0, "RobotDriveDevRef"=w331) -> ("error out"=w330:errorcluster)  [unwired: 4 in, 2 out]
              n212 = call "Drive Back9"("error in (no error)"=w330, "Delay Time (s)"=2.0) -> ("error out"=w266:errorcluster)  [unwired: 9 in]
              n213 = call <vilib>:"WPI_RobotDriveRefNum Registry Get.vi"("error in (no error)"=w266, "refnum name"="LiftMotors") -> ("error out"=w341:errorcluster, "RobotDriveDevRef"=w343:T3)  [unwired: 8 in]
              n214 = call-poly <vilib>:"WPI_RobotDriveArcadeDrive.vi"("error in (no error)"=w341, "Y axis value"=-30.0, "X axis value"=0.0 ("X"), "RobotDriveDevRef"=w343) -> ("error out"=w344:errorcluster)  [unwired: 5 in, 2 out]
              n215 = call "Drop Tote9"("error in (no error)"=w344, "Delay Time (s)"=0.5) -> ()  [unwired: 9 in, 1 out]
            }
            frame Enabled {
            }
          }
        }
      }
    }
  }
  "?" <- "Can you find me?"
